vi "Set Shared Memory Size.vi"(8 "error in (no error)":errorcluster, 10 "size (bytes)":u32, 11 "shared memory in":T1) -> (0 "error out":errorcluster, 3 "shared memory out":T1)   [LabVIEW 2013, in "Linux RT IPC.lvlib" / "Shared Memory.lvlib" / "Shared Memory.lvclass"]
doc: "This VI allows the size of the shared memory file to be set to a certain number of bytes. Memory operations are more efficient when the allocated memory is some multiple of the system page size. Use this VI in conjunction with the Get System Page Size VI to set the size of the shared memory to be a multiple of the page size."
uses:
  Shared Memory.lvclass
  Controls/reference.ctl
  Shared Memory.lvclass/Shared Memory.ctl
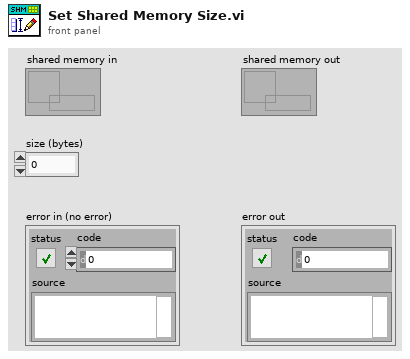
[diagram p1: front panel]
types:
  T1 = typedef "Linux RT IPC.lvlib/Shared Memory.lvlib/Shared Memory.lvclass/reference.ctl" = refnum<data-value>
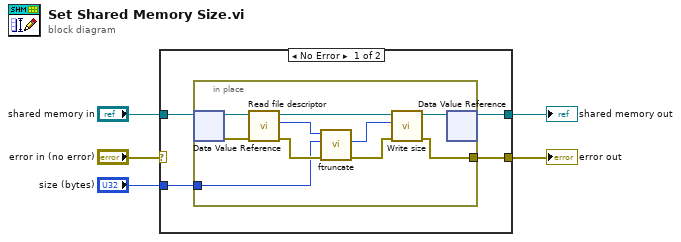
[diagram p0: block diagram]
diagram:
  n1 = case shown="No Error" "error in (no error)" {
    selector: "error in (no error)" -> [_ w20]
    tunnel: "shared memory in" -> [w9 w21]
    tunnel: [w8 w20] -> w2
    tunnel: [w7 w21] -> w4
    tunnel: "size (bytes)" -> [w6 _]
    frame No Error {
      n2 = in-place {
        in-place-border: [w11] -> w8
        in-place-border: w6 -> [w10]
        n3 = in-place-dvr #1(w9) -> (w14:refnum<class "Shared Memory.lvclass">, w12:errorcluster)
        n4 = call "Read file descriptor.vi"("error in (no error)"=w12, "Shared Memory in"=w14) -> ("error out"=w17:errorcluster, "file descriptor"=w16:i32, "Shared Memory out"=w15:refnum<class "Shared Memory.lvclass">)  [unwired: 7 in]
        n5 = call "ftruncate.vi"("error in (no error)"=w17, "size (bytes)"=w10, "file descriptor"=w16) -> ("error out"=w19:errorcluster, "size (bytes)"=w18:u32)  [unwired: 6 in, 1 out]
        n6 = call "Write size.vi"("error in (no error)"=w19, "size (bytes)"=w18, "Shared Memory in"=w15) -> ("error out"=w11:errorcluster, "Shared Memory out"=w13:refnum<class "Shared Memory.lvclass">)  [unwired: 7 in]
        n7 = in-place-dvr #1(w13) -> (w7:T1)  [unwired: 1 out]
      }
    }
    frame Error {
    }
  }
  "error out" <- w2
  "shared memory out" <- w4
